vi "Periodic Tasks.vi"(8 "error in":errorcluster) -> ()   [LabVIEW 2017]
doc: "This VI runs in parallel to other tasks. It can contain as many user-defined periodic loops as you need. These can carry out PID or other sorts of timed response."
uses:
  <vilib>/Rock Robotics/WPI/ThirdParty/Sensors/navX/_TypeDefs/FRIC_navX_DeviceNumbersTypeDef.ctl
  <vilib>/Rock Robotics/WPI/Utilities/WPI_GetSetVariantRefNum.vi
  Robot Global Data.vi
  <vilib>/Rock Robotics/Network Tables/NT Read Boolean.vi
  <vilib>/Rock Robotics/Network Tables/NT Write Boolean.vi
  <vilib>/Rock Robotics/Network Tables/NT Write Number.vi
  Lift States.ctl
  <vilib>/Rock Robotics/WPI/DriverStation/WPI_DriverStationAllianceInfo.ctl
panel:
  in  "Lift Max Value":dbl=800.0
  in  "Red Alliance":bool
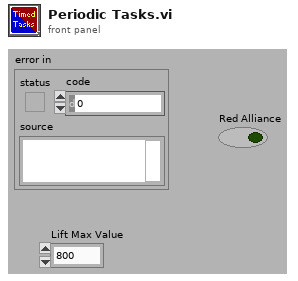
[diagram p1: front panel]
types:
  T1 = typedef "WPI_DriverStationAllianceInfo.ctl" = enum16{"Red", "Blue", "Invalid"}
  T2 = typedef "Lift States.ctl" = enum16{"Manual", "Scale Low", "Scale Middle", "Scale High", "Rock Bottom", "Almost Down"}
  T3 = typedef "WPI_I2CDevRef.ctl" = cluster{"DevStatus":errorcluster, "Device Address":u8, "Handle":i32, "I2C Bus":T4}
  T4 = typedef "i2c_bus.ctl" = enum16{"I2C On-Board", "I2C MXP", "Invalid"}
  T5 = typedef "WPI_MotorControlDeviceRef.ctl" = cluster{"DeviceStatus":errorcluster, "Type":T6, "PWM":cluster{"PWM Channel":T7, "DeadBand":T8}, "CAN":cluster{"Device Number":u8, "SetOutput VI Ref":variant, "GetOutput VI Ref":variant, "Enable VI Ref":variant, "Disable VI Ref":variant, "Data":variant}, "Invert":bool, "DIO PWM":cluster{"PWM \"Enable\" Channel":T7, "DIOChannel":T9, "PWM Rate":dbl}}
  T6 = typedef "WPI_MotorControlType.ctl" = enum16{"PWM", "CAN", "DIO PWM"}
  T7 = typedef "FPGA_DIOPWMChannel.ctl" = enum8{"PWM 0", "PWM 1", "PWM 2", "PWM 3", "PWM 4", "PWM 5", "PWM 6", "PWM 7", "PWM 8", "PWM 9", "PWM MXP 0", "PWM MXP 1", "PWM MXP 2", "PWM MXP 3", "PWM MXP 4", "PWM MXP 5", "PWM MXP 6", "PWM MXP 7", "PWM MXP 8", "PWM MXP 9", "Invalid"}
  T8 = typedef "WPI_PWMDeadband.ctl" = cluster{"Name":string, "maxPositivePwm":i32, "minPositivePwm":i32, "centerPwm":i32, "maxNegativePwm":i32, "minNegativePwm":i32, "angularRange":u16}
  T9 = typedef "FPGA_DIOChannel.ctl" = enum8{"DIO 0", "DIO 1", "DIO 2", "DIO 3", "DIO 4", "DIO 5", "DIO 6", "DIO 7", "DIO 8", "DIO 9", "DIO MXP 0", "DIO MXP 1", "DIO MXP 2", "DIO MXP 3", "DIO MXP 4", "DIO MXP 5", "DIO MXP 6", "DIO MXP 7", "DIO MXP 8", "DIO MXP 9", "DIO MXP 10", "DIO MXP 11", "DIO MXP 12", "DIO MXP 13", "DIO MXP 14", "DIO MXP 15", "SPI Port CS1", "SPI Port CS2", "SPI Port CS3", "SPI Port MISO", "SPI Port MOSI", "Invalid"}
  T10 = typedef "WPI_SolenoidDevRef.ctl" = cluster{"DevStatus":errorcluster, "Pneumatics Control Module":u8, "Forward Solenoid Channel":T11, "Reverse Solenoid Channel":T11}
  T11 = typedef "WPI_SolenoidChannel.ctl" = enum8{"Solenoid 0", "Solenoid 1", "Solenoid 2", "Solenoid 3", "Solenoid 4", "Solenoid 5", "Solenoid 6", "Solenoid 7", "Invalid"}
  T12 = typedef "WPI_JoystickDevRef.ctl" = cluster{"Device":T13}
  T13 = typedef "WPI_JoystickDeviceEnum.ctl" = enum16{"USB 0", "USB 1", "USB 2", "USB 3", "USB 4", "USB 5"}
  T14 = cluster{"MotorControlDevRef":T5, "MotorControlDevRef":T5, "SolenoidDevRef":T10, "MotorControlDevRef":T5, "MotorControlDevRef":T5, "MotorControlDevRef":T5, "MotorControlDevRef":T5, "MotorControlDevRef":T5, "SolenoidDevRef":T10}
  T15 = cluster{"JoystickDevRef":T12, "JoystickDevRef":T12, "JoystickDevRef":T12, "JoystickDevRef":T12}
  T16 = typedef "WPI_EncoderDevRef.ctl" = cluster{"DevStatus":errorcluster, "EncoderIndex":T17, "CounterIndex":T18, "DistancePerCount":dbl, "Decoding Type":T19}
  T17 = typedef "FPGA_EncoderIdx.ctl" = enum8{"Enc 0", "Enc 1", "Enc 2", "Enc 3", "Enc 4", "Enc 5", "Enc 6", "Enc 7", "Invalid"}
  T18 = typedef "FPGA_CounterCtrSystemIndex.ctl" = enum8{"Ctr 0", "Ctr 1", "Ctr 2", "Ctr 3", "Ctr 4", "Ctr 5", "Ctr 6", "Ctr 7", "Invalid"}
  T19 = typedef "WPI_EncoderType.ctl" = enum16{"1x", "2x", "4x"}
  T20 = cluster{"EncoderDevRef":T16, "EncoderDevRef":T16}
  T21 = typedef "FRIC_navX_DeviceNumbersTypeDef.ctl" = enum16{"Dev0", "Dev1", "Dev2", "Dev3"}
  T22 = cluster{"Yaw":dbl, "Roll":dbl, "Pitch":dbl, "Heading":dbl, "Fused Heading":dbl}
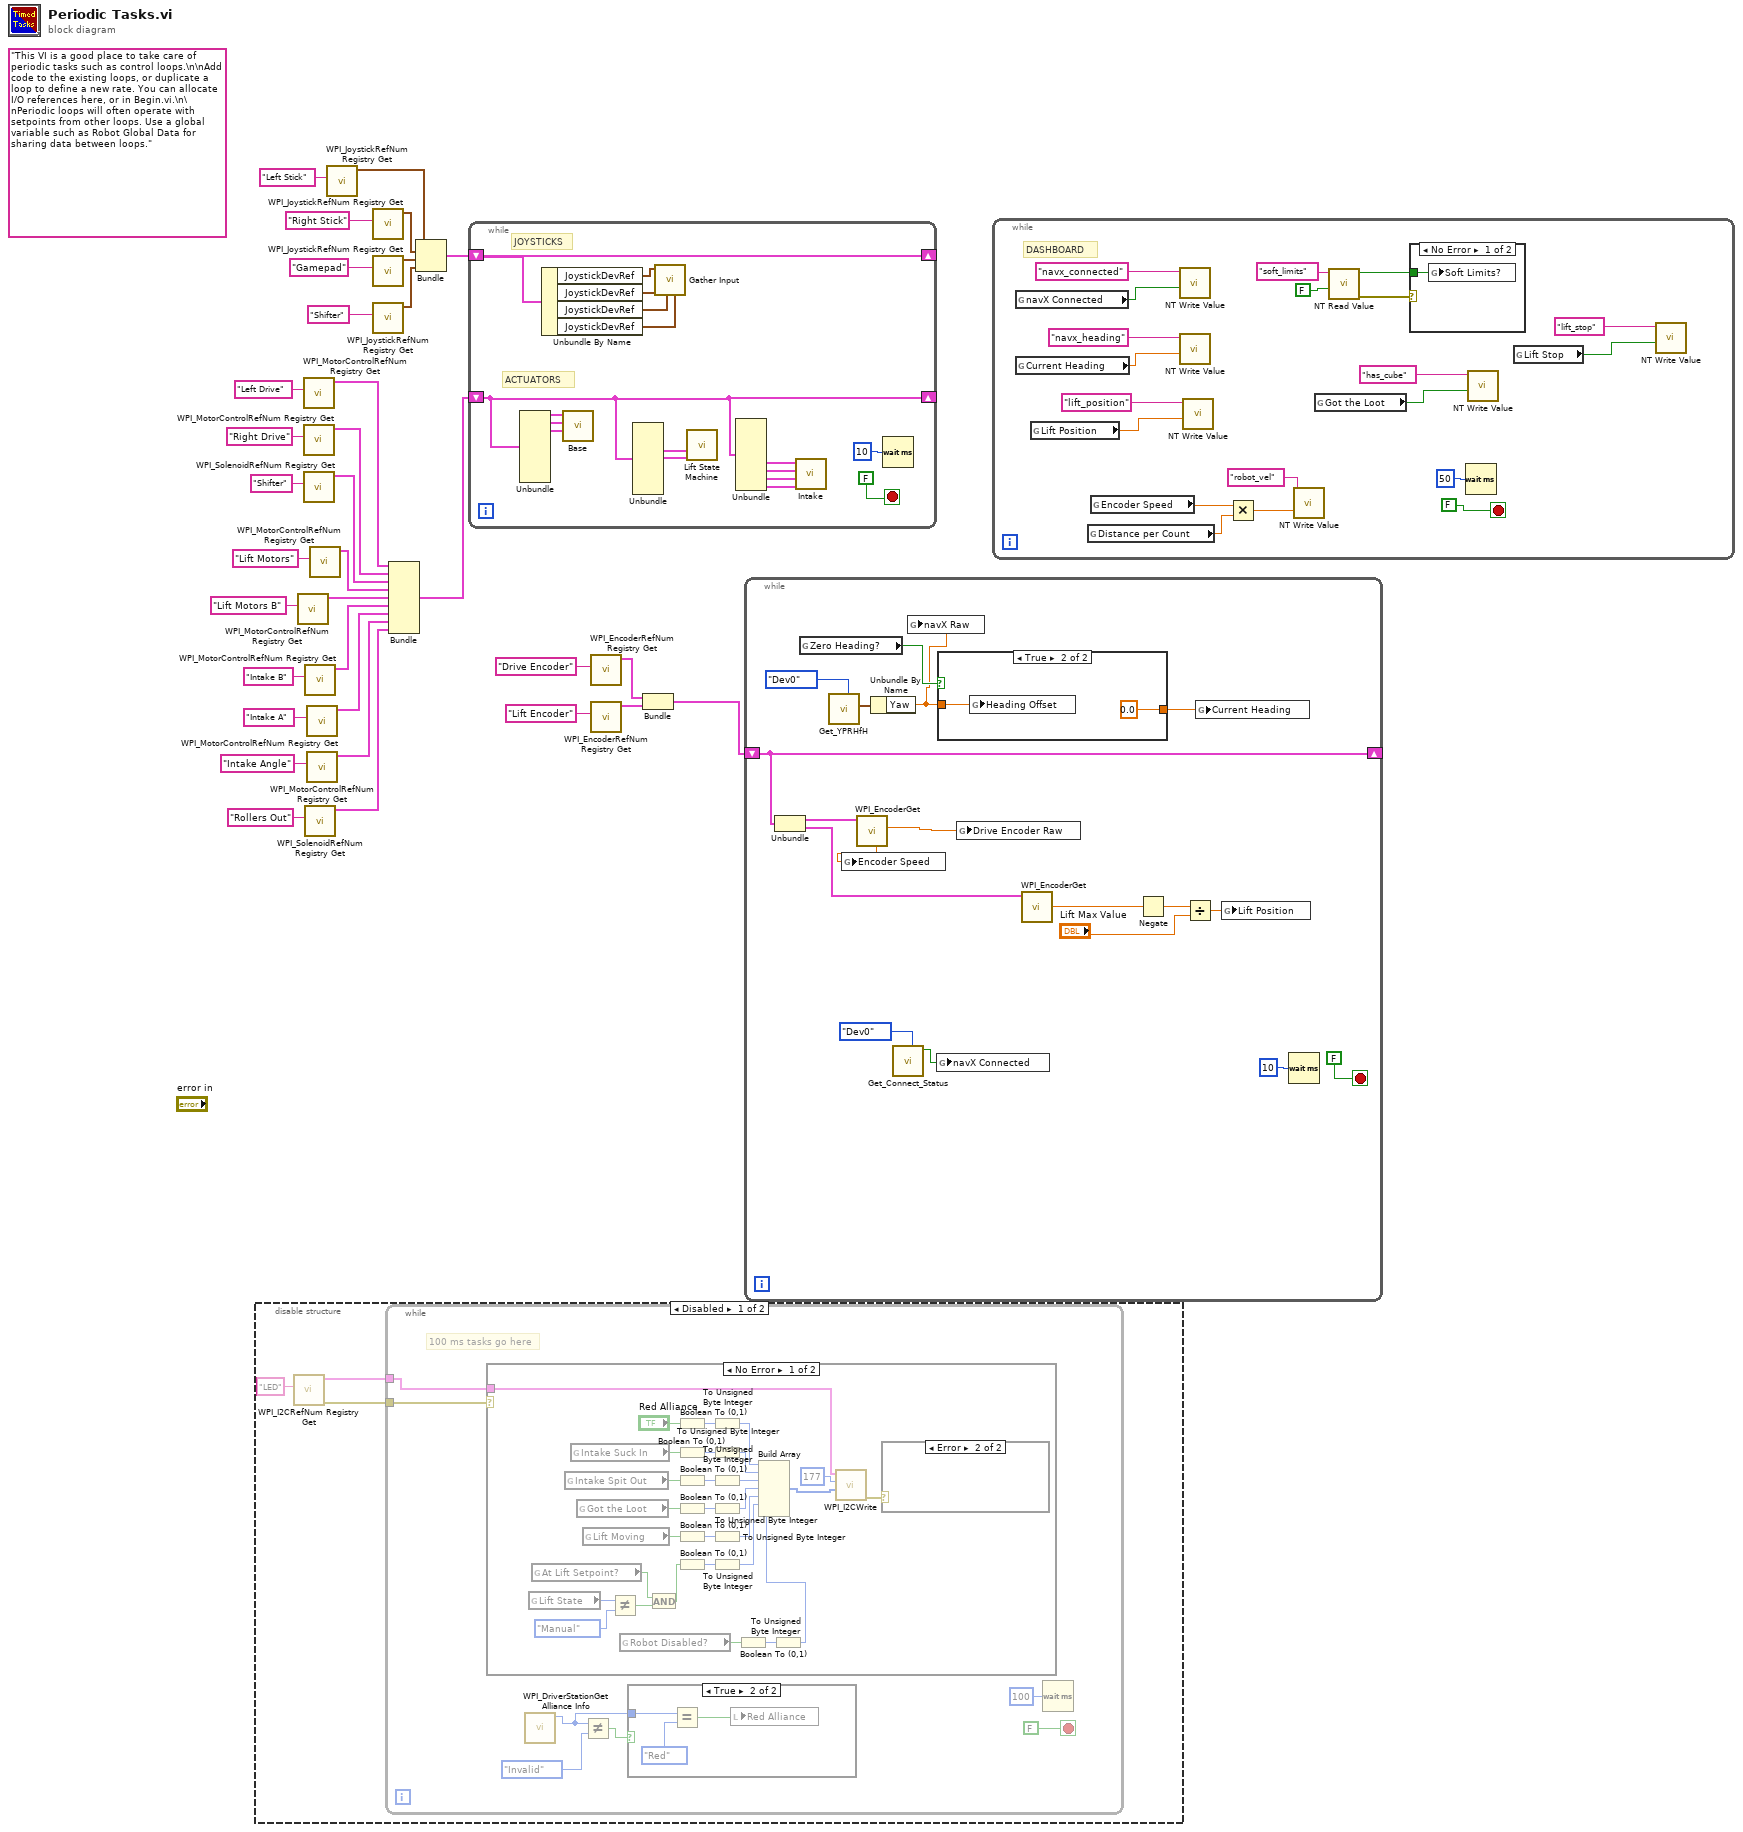
[diagram p0: block diagram]
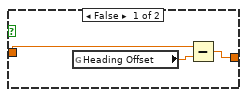
[diagram p7: hidden frame]
diagram:
  (unwired) "This VI is a good place to take care of periodic tasks such as control loops.\n\nAdd code to the existing loops, or duplicate a loop to define a new rate. You can allocate I/O references here, or in Begin.vi.\n\nPeriodic loops will often operate with setpoints from other loops. Use a global variable such as Robot Global Data for sharing data between loops."
  n1 = disable-structure shown="Disabled" {
    frame Disabled {
      n2 = call <vilib>:"WPI_I2CRefNum Registry Get.vi"("refnum name"="LED") -> ("error out"=w34:errorcluster, "I2CDevRef"=w35:T3)  [unwired: 9 in]
      n3 = while {
        tunnel: w35 -> [w40]
        tunnel: w34 -> [w41]
        stop <- FALSE stop-if-true
        # "100 ms tasks go here"
        n4 = case shown="No Error" w41 {
          tunnel: w40 -> [w71 _]
          frame No Error {
            n5 = global read "Robot Global Data.vi" "Lift State"() -> (w54:T2)
            n6 = global read "Robot Global Data.vi" "At Lift Setpoint?"() -> (w51:bool)
            n7 = global read "Robot Global Data.vi" "Intake Spit Out"() -> (w61:bool)
            n8 = global read "Robot Global Data.vi" "Intake Suck In"() -> (w60:bool)
            n9 = global read "Robot Global Data.vi" "Got the Loot"() -> (w62:bool)
            n10 = global read "Robot Global Data.vi" "Lift Moving"() -> (w57:bool)
            n11 = Not Equal?(x=w54, y=Lift_States."Manual") -> (x != y?=w50:bool)
            n12 = global read "Robot Global Data.vi" "Robot Disabled?"() -> (w49:bool)
            n13 = And(x=w51, y=w50) -> (x .and. y?=w52:bool)
            n14 = Boolean To (0,1)(Boolean="Red Alliance") -> (0, 1=w68:i16)
            n15 = Boolean To (0,1)(Boolean=w60) -> (0, 1=w67:i16)
            n16 = Boolean To (0,1)(Boolean=w61) -> (0, 1=w66:i16)
            n17 = Boolean To (0,1)(Boolean=w62) -> (0, 1=w65:i16)
            n18 = Boolean To (0,1)(Boolean=w57) -> (0, 1=w59:i16)
            n19 = Boolean To (0,1)(Boolean=w52) -> (0, 1=w56:i16)
            n20 = To Unsigned Byte Integer(number=w68) -> (unsigned 8bit integer=w75:u8)
            n21 = To Unsigned Byte Integer(number=w67) -> (unsigned 8bit integer=w74:u8)
            n22 = To Unsigned Byte Integer(number=w66) -> (unsigned 8bit integer=w64:u8)
            n23 = To Unsigned Byte Integer(number=w65) -> (unsigned 8bit integer=w63:u8)
            n24 = To Unsigned Byte Integer(number=w59) -> (unsigned 8bit integer=w58:u8)
            n25 = To Unsigned Byte Integer(number=w56) -> (unsigned 8bit integer=w55:u8)
            n26 = Boolean To (0,1)(Boolean=w49) -> (0, 1=w48:i16)
            n27 = To Unsigned Byte Integer(number=w48) -> (unsigned 8bit integer=w47:u8)
            n28 = Build Array(w75, w74, w64, w63, w58, w55, w47) -> (w73:u8[])
            n29 = call <vilib>:"WPI_I2CWrite.vi"("I2CDataToSend"=w73, "I2CRegister"=u8 177, "I2CDevRef"=w71) -> ("error out"=w70:errorcluster)  [unwired: 7 in, 1 out]
            n30 = case shown="Error" w70 {
              frame No Error {
              }
              frame Error {
              }
            }
          }
          frame Error {
          }
        }
        n31 = call <vilib>:"WPI_DriverStationGet Alliance Info.vi"() -> ("Alliance"=w37:T1)  [unwired: 6 in, 5 out]
        n32 = Not Equal?(x=w37, y=WPI_DriverStationAllianceInfo."Invalid") -> (x != y?=w38:bool)
        n33 = case shown="True" w38 {
          tunnel: w37 -> [_ w46]
          frame False {
          }
          frame True {
            n34 = Equal?(x=w46, y=WPI_DriverStationAllianceInfo."Red" ("x")) -> (x = y?=w44:bool)
            n35 = local write "Red Alliance"(w44) -> ()
          }
        }
        n36 = Wait (ms)(milliseconds to wait=u32 100) -> ()  [unwired: 1 out]
      }
    }
    frame Enabled {
    }
  }
  n37 = call <vilib>:"WPI_MotorControlRefNum Registry Get.vi"("refnum name"="Lift Motors B") -> ("MotorControlDevRef"=w18:T5)  [unwired: 9 in, 1 out]
  n38 = call <vilib>:"WPI_MotorControlRefNum Registry Get.vi"("refnum name"="Left Drive") -> ("MotorControlDevRef"=w30:T5)  [unwired: 9 in, 1 out]
  n39 = call <vilib>:"WPI_MotorControlRefNum Registry Get.vi"("refnum name"="Right Drive") -> ("MotorControlDevRef"=w29:T5)  [unwired: 9 in, 1 out]
  n40 = call <vilib>:"WPI_SolenoidRefNum Registry Get.vi"("refnum name"="Shifter") -> ("SolenoidDevRef"=w24:T10)  [unwired: 9 in, 1 out]
  n41 = call <vilib>:"WPI_MotorControlRefNum Registry Get.vi"("refnum name"="Intake B") -> ("MotorControlDevRef"=w26:T5)  [unwired: 9 in, 1 out]
  n42 = call <vilib>:"WPI_SolenoidRefNum Registry Get.vi"("refnum name"="Rollers Out") -> ("SolenoidDevRef"=w20:T10)  [unwired: 9 in, 1 out]
  n43 = call <vilib>:"WPI_MotorControlRefNum Registry Get.vi"("refnum name"="Intake A") -> ("MotorControlDevRef"=w3:T5)  [unwired: 9 in, 1 out]
  n44 = call <vilib>:"WPI_MotorControlRefNum Registry Get.vi"("refnum name"="Intake Angle") -> ("MotorControlDevRef"=w1:T5)  [unwired: 9 in, 1 out]
  n45 = call <vilib>:"WPI_MotorControlRefNum Registry Get.vi"("refnum name"="Lift Motors") -> ("MotorControlDevRef"=w23:T5)  [unwired: 9 in, 1 out]
  n46 = call <vilib>:"WPI_JoystickRefNum Registry Get.vi"("refnum name"="Left Stick") -> ("JoystickDevRef"=w13:T12)  [unwired: 9 in, 1 out]
  n47 = call <vilib>:"WPI_JoystickRefNum Registry Get.vi"("refnum name"="Right Stick") -> ("JoystickDevRef"=w12:T12)  [unwired: 9 in, 1 out]
  n48 = call <vilib>:"WPI_JoystickRefNum Registry Get.vi"("refnum name"="Gamepad") -> ("JoystickDevRef"=w11:T12)  [unwired: 9 in, 1 out]
  n49 = call <vilib>:"WPI_JoystickRefNum Registry Get.vi"("refnum name"="Shifter") -> ("JoystickDevRef"=w10:T12)  [unwired: 9 in, 1 out]
  n50 = Bundle("MotorControlDevRef"=w30, "MotorControlDevRef"=w29, "SolenoidDevRef"=w24, "MotorControlDevRef"=w23, "MotorControlDevRef"=w18, "MotorControlDevRef"=w26, "MotorControlDevRef"=w3, "MotorControlDevRef"=w1, "SolenoidDevRef"=w20) -> (w9:T14)  [unwired: 1 in]
  n51 = Bundle("JoystickDevRef"=w13, "JoystickDevRef"=w12, "JoystickDevRef"=w11, "JoystickDevRef"=w10) -> (w33:T15)  [unwired: 1 out]
  n52 = while {
    shift-right: [w90] -> _
    shift-left: w33 -> [w90]
    shift-right: [w85] -> _
    shift-left: w9 -> [w85]
    stop <- FALSE stop-if-true
    # "JOYSTICKS"
    # "ACTUATORS"
    n53 = Unbundle(w85) -> ("MotorControlDevRef"=w84:T5, "MotorControlDevRef"=w83:T5, "SolenoidDevRef"=w82:T10)  [unwired: 6 out]
    n54 = Unbundle By Name(w90) -> ("JoystickDevRef"=w89:T12, "JoystickDevRef"=w88:T12, "JoystickDevRef"=w86:T12, "JoystickDevRef"=w87:T12)
    n55 = call "Base.vi"("Shifter"=w82, "Right Drive"=w83, "Left Drive"=w84) -> ()  [unwired: 9 in]
    n56 = Unbundle(w85) -> ("MotorControlDevRef"=w80:T5, "MotorControlDevRef"=w78:T5)  [unwired: 7 out]
    n57 = call "Gather Input.vi"("Shifter"=w87, "Gamepad"=w86, "Joystick Right"=w88, "Joystick Left"=w89) -> ()  [unwired: 8 in]
    n58 = call "Lift State Machine.vi"("Lift Motors B"=w78, "Lift Motors"=w80) -> ()  [unwired: 10 in]
    n59 = Unbundle(w85) -> ("MotorControlDevRef"=w81:T5, "MotorControlDevRef"=w76:T5, "MotorControlDevRef"=w77:T5, "SolenoidDevRef"=w79:T10)  [unwired: 5 out]
    n60 = call "Intake.vi"("Rollers Out"=w79, "Intake Angle"=w77, "Motor A"=w76, "Motor B"=w81) -> ()  [unwired: 8 in]
    n61 = Wait (ms)(milliseconds to wait=u32 10) -> ()  [unwired: 1 out]
  }
  n62 = call <vilib>:"WPI_EncoderRefNum Registry Get.vi"("refnum name"="Drive Encoder") -> ("EncoderDevRef"=w8:T16)  [unwired: 9 in, 1 out]
  n63 = call <vilib>:"WPI_EncoderRefNum Registry Get.vi"("refnum name"="Lift Encoder") -> ("EncoderDevRef"=w6:T16)  [unwired: 9 in, 1 out]
  n64 = Bundle("EncoderDevRef"=w8, "EncoderDevRef"=w6) -> (w7:T20)  [unwired: 1 in]
  n65 = while {
    shift-right: [w105] -> _
    shift-left: w7 -> [w105]
    stop <- FALSE stop-if-true
    n66 = Unbundle(w105) -> ("EncoderDevRef"=w104:T16, "EncoderDevRef"=w94:T16)
    n67 = global read "Robot Global Data.vi" "Zero Heading?"() -> (w110:bool)
    n68 = call <vilib>:"Get_YPRHfH.vi"("Device Number"=FRIC_navX_DeviceNumbersTypeDef."Dev0") -> ("YRPHfH"=w109:T22)  [unwired: 10 in]
    n69 = call <vilib>:"WPI_EncoderGet.vi"("EncoderDevRef"=w104) -> ("Distance"=w93:dbl, "Rate"=w99:dbl)  [unwired: 5 in, 4 out]
    n70 = global write "Robot Global Data.vi" "Encoder Speed"(w99) -> ()
    n71 = Unbundle By Name(w109) -> ("Yaw"=w100:dbl)
    n72 = call <vilib>:"Get_Connect_Status.vi"("Device Number"=FRIC_navX_DeviceNumbersTypeDef."Dev0") -> ("Connected"=w101:bool)  [unwired: 10 in]
    n73 = global write "Robot Global Data.vi" "navX Raw"(w100) -> ()
    n74 = global write "Robot Global Data.vi" "navX Connected"(w101) -> ()
    n75 = case shown="True" w110 {
      tunnel: w100 -> [w113 w115]
      tunnel: [w111 0.0] -> w108
      frame False {
        n76 = global read "Robot Global Data.vi" "Heading Offset"() -> (w112:dbl)
        n77 = Subtract(x=w113, y=w112) -> (x-y=w111:dbl)
      }
      frame True {
        n78 = global write "Robot Global Data.vi" "Heading Offset"(w115) -> ()
      }
    }
    n79 = global write "Robot Global Data.vi" "Drive Encoder Raw"(w93) -> ()
    n80 = call <vilib>:"WPI_EncoderGet.vi"("EncoderDevRef"=w94) -> ("Distance"=w96:dbl)  [unwired: 5 in, 5 out]
    n81 = Negate(x=w96) -> (-x=w95:dbl)
    n82 = Divide(x=w95, y="Lift Max Value") -> (x/y=w97:dbl)
    n83 = global write "Robot Global Data.vi" "Current Heading"(w108) -> ()
    n84 = global write "Robot Global Data.vi" "Lift Position"(w97) -> ()
    n85 = Wait (ms)(milliseconds to wait=u32 10) -> ()  [unwired: 1 out]
  }
  n86 = while {
    stop <- FALSE stop-if-true
    # "DASHBOARD"
    n87 = global read "Robot Global Data.vi" "navX Connected"() -> (w133:bool)
    n88 = global read "Robot Global Data.vi" "Current Heading"() -> (w131:dbl)
    n89 = global read "Robot Global Data.vi" "Lift Position"() -> (w129:dbl)
    n90 = global read "Robot Global Data.vi" "Distance per Count"() -> (w119:dbl)
    n91 = global read "Robot Global Data.vi" "Encoder Speed"() -> (w118:dbl)
    n92 = call-poly <vilib>:"NT Write Value.vi"("Boolean"=w133, "Name"="navx_connected") -> ()  [unwired: 9 in, 1 out]
    n93 = call-poly <vilib>:"NT Write Value.vi"("Numeric"=w131, "Name"="navx_heading") -> ()  [unwired: 9 in, 1 out]
    n94 = call-poly <vilib>:"NT Write Value.vi"("Numeric"=w129, "Name"="lift_position") -> ()  [unwired: 9 in, 1 out]
    n95 = Multiply(x=w118, y=w119) -> (x*y=w120:dbl)
    n96 = call-poly <vilib>:"NT Write Value.vi"("Numeric"=w120, "Name"="robot_vel") -> ()  [unwired: 9 in, 1 out]
    n97 = global read "Robot Global Data.vi" "Got the Loot"() -> (w122:bool)
    n98 = call-poly <vilib>:"NT Read Value.vi"("Default Value"=FALSE, "Name"="soft_limits") -> ("error out"=w125:errorcluster, "Boolean"=w124:bool)  [unwired: 8 in]
    n99 = case shown="No Error" w125 {
      tunnel: w124 -> [w136 _]
      frame No Error {
        n100 = global write "Robot Global Data.vi" "Soft Limits?"(w136) -> ()
      }
      frame Error {
      }
    }
    n101 = Wait (ms)(milliseconds to wait=u32 50) -> ()  [unwired: 1 out]
    n102 = call-poly <vilib>:"NT Write Value.vi"("Boolean"=w122, "Name"="has_cube") -> ()  [unwired: 9 in, 1 out]
    n103 = global read "Robot Global Data.vi" "Lift Stop"() -> (w117:bool)
    n104 = call-poly <vilib>:"NT Write Value.vi"("Boolean"=w117, "Name"="lift_stop") -> ()  [unwired: 9 in, 1 out]
  }
